vi "Opgave 5 Lige Ulige.vi"(11 "Antal tilfældige tal":u64) -> (0 "Lige":u64[](array[numeric]), 1 "Flest ulige":bool, 2 "Flest Lige":bool, 3 "Samme antal":bool, 4 "Ulige":u64[](array[numeric]))   [LabVIEW 2019]
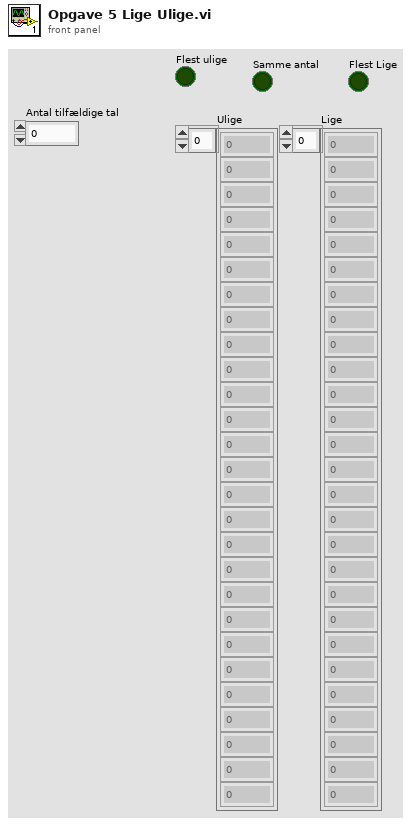
[diagram p1: front panel]
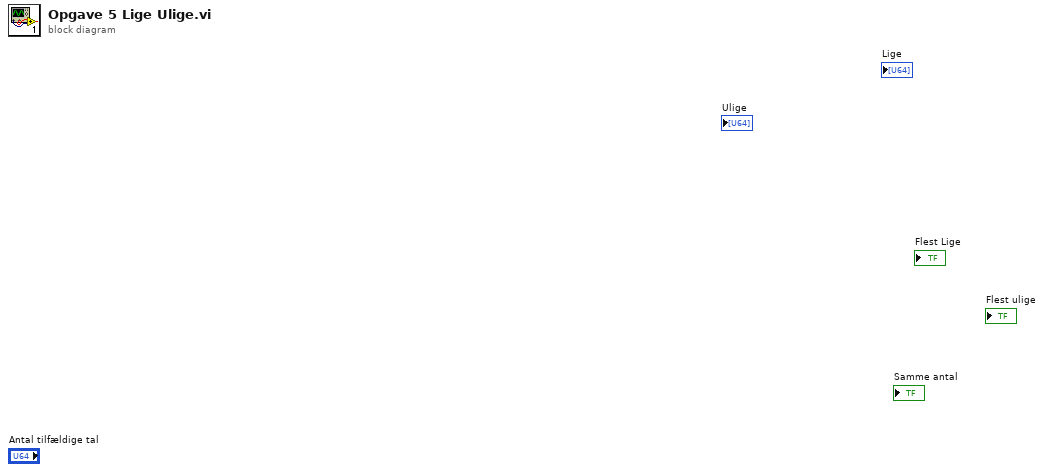
[diagram p0: block diagram]
diagram:
